vi "Word (Frame).vi"(8 "error in (no error)":errorcluster, 11 "Node Ptr":T2 format="%.0x") -> (0 "error out":errorcluster)   [LabVIEW 2020, in "Communication Bus Template System Explorer.lvlib" / "Implementation.lvlib"]
uses:
  Implementation.lvlib
  <vilib>/NI VeriStand/Custom Device API/Custom Device Item Ref.ctl
  <vilib>/NI VeriStand/Custom Device API/Custom Device API.lvlib
  Scripting/Communication Bus Template Scripting.lvlib
  Scripting/Constants.vi
  <vilib>/NI VeriStand/Custom Device API/Get Item Property (U16).vi
  <vilib>/NI VeriStand/Custom Device API/Get Item Property (Double).vi
  <vilib>/NI VeriStand/Custom Device API/Get Item Property (U32).vi
  <vilib>/NI VeriStand/Custom Device API/Get Item Property (Boolean).vi
panel:
  out "Transfer Type":T1(ring)
  out "SDI":u8 format="%o"
  out "SDI Enabled":bool
  out "Transfer Rate (Hz)":dbl
  out "Label (Octal)":i32 format="%o"
  out "Label (Decimal)":i32
  in  "SHDocVw.IWebBrowser":refnum<k7>(container)
  in  "Specific Header":cluster{"Section Name":string}={"Section Name"="Specific Page Settings"}
  in  "General Header":cluster{"Section Name":string}={"Section Name"="General Page Settings"}
  in  "Description":string
  in  "Name":string
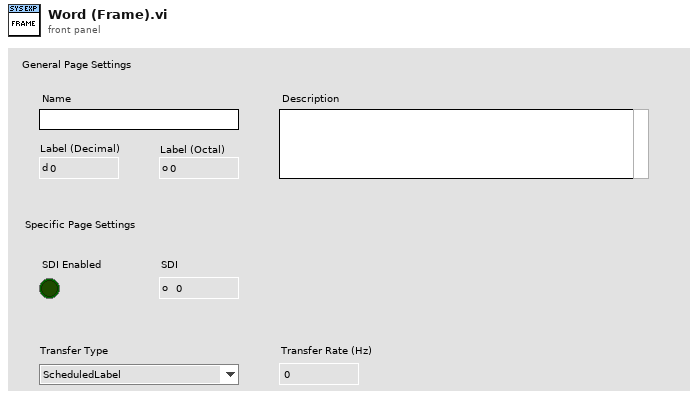
[diagram p1: front panel]
types:
  T1 = enum16{"ScheduledLabel", "Acyclic", "Block", "Strobe"}
  T2 = typedef "Custom Device API.lvlib/Custom Device Item Ref.ctl" = u64
  T3 = typedef "Custom Device API.lvlib/Custom Device Item Info.ctl" = cluster{"Name":string, "Is Channel":bool, "GUID":string, "Is Waveform":bool}
  T4 = typedef "Custom Device API.lvlib/Custom Device Commands.ctl" = enum16{"Default", "Item renamed", "Shutdown", "Dynamic button pressed"}
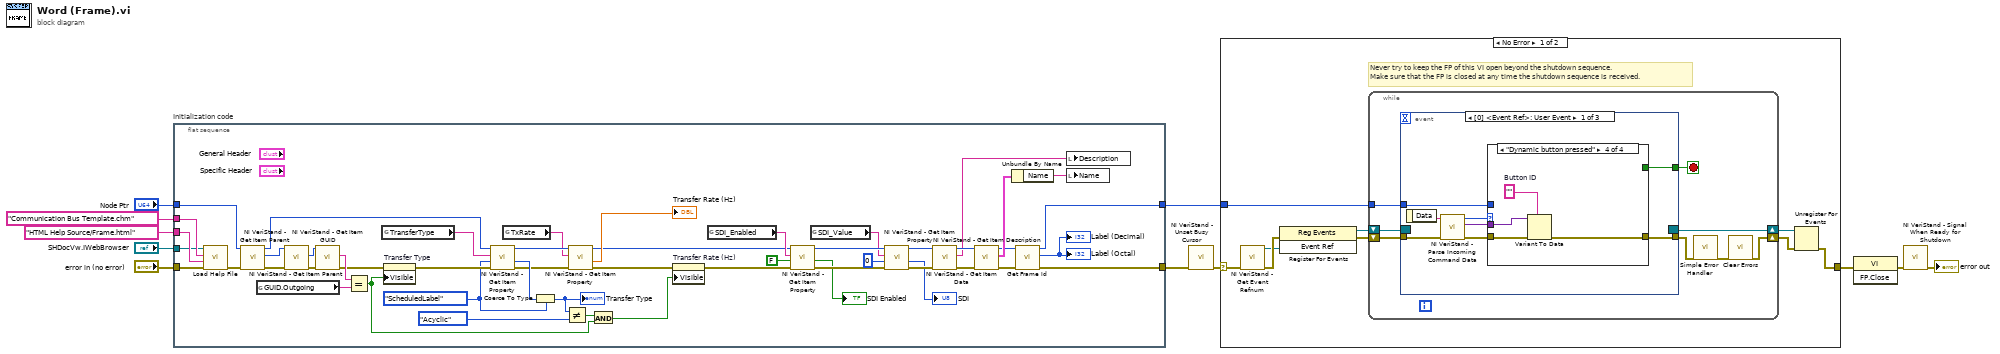
[diagram p0: block diagram]
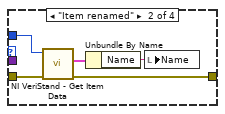
[diagram p3: hidden frame]
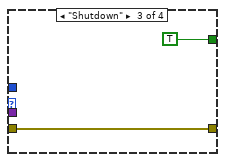
[diagram p4: hidden frame]
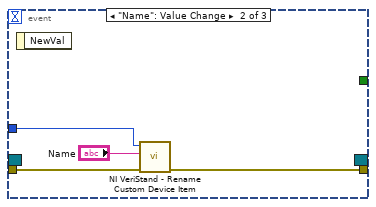
[diagram p5: hidden frame]
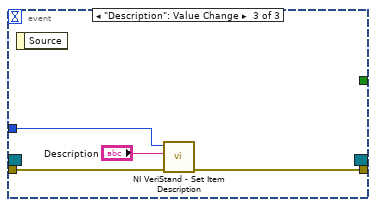
[diagram p6: hidden frame]
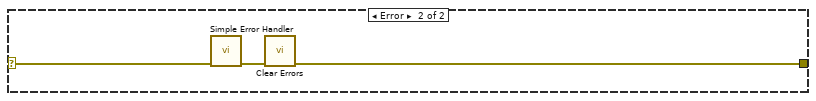
[diagram p7: hidden frame]
diagram:
  n1 = flat-sequence "Initialization code" {
    tunnel: "error in (no error)" -> [w55]
    tunnel: "Node Ptr" -> [w40]
    tunnel: [w49] -> w7
    tunnel: [w48] -> w4
    tunnel: "SHDocVw.IWebBrowser" -> [w52]
    tunnel: "HTML Help Source/Frame.html" ("CD_CHM_Section") -> [w54]
    tunnel: "Communication Bus Template.chm" ("CD_CHM_FileName") -> [w53]
    frame #0 {
      w35 = T1."ScheduledLabel" ("Transfer Type")
      n2 = call "Load Help File.vi"("error in (no error)"=w55, "HTML File to Load"=w54, "Main CHM File"=w53, "Browser"=w52) -> ("error out"=w41:errorcluster)  [unwired: 7 in]
      n3 = call <vilib>:"NI VeriStand - Get Item Parent.vi"("error in (no error)"=w41, "Item Ref in"=w40) -> ("error out"=w46:errorcluster, "Parent Ref"=w45:T2, "Item Ref out"=w36:T2)  [unwired: 6 in, 1 out]
      n4 = global read "Constants.vi" "GUID.Outgoing"() -> (w39:string)
      n5 = call <vilib>:"NI VeriStand - Get Item Parent.vi"("error in (no error)"=w46, "Item Ref in"=w45) -> ("error out"=w44:errorcluster, "Parent Ref"=w42:T2)  [unwired: 6 in, 2 out]
      n6 = call <vilib>:"NI VeriStand - Get Item GUID.vi"("error in (no error)"=w44, "Item Ref in"=w42) -> ("error out"=w38:errorcluster, "GUID"=w43:string)  [unwired: 7 in, 1 out]
      n7 = Equal?(x=w43, y=w39) -> (x = y?=w30:bool)
      n8 = global read "Constants.vi" "TransferType"() -> (w28:string)
      n9 = property on="Transfer Type" class="Enum (strict)"(error in=w38, "Visible"=w30) -> (error out=w37:errorcluster)  [unwired: 1 in, 1 out]
      n10 = call-poly <vilib>:"NI VeriStand - Get Item Property.vi"("error in (no error)"=w37, "Default Value"=w35, "Property Name"=w28, "Item Ref in"=w36) -> ("error out"=w27:errorcluster, "Value"=w34:u16, "Item Ref out"=w25:T2)  [unwired: 4 in, 1 out]
      n11 = global read "Constants.vi" "TxRate"() -> (w24:string)
      n12 = Coerce To Type(0:w34, 1:w35) -> (2:w33:T1)
      "Transfer Type" <- w33
      n13 = Not Equal?(x=w33, y=T1."Acyclic" ("Transfer Type")) -> (x != y?=w31:bool)
      n14 = call-poly <vilib>:"NI VeriStand - Get Item Property.vi"("error in (no error)"=w27, "Property Name"=w24, "Item Ref in"=w25) -> ("error out"=w26:errorcluster, "Value"=→"Transfer Rate (Hz)":dbl, "Item Ref out"=w17:T2)  [unwired: 5 in, 1 out]
      n15 = And(x=w31, y=w30) -> (x .and. y?=w29:bool)
      n16 = property on="Transfer Rate (Hz)" class="DigNum (strict)"(error in=w26, "Visible"=w29) -> (error out=w16:errorcluster)  [unwired: 1 in, 1 out]
      n17 = global read "Constants.vi" "SDI_Enabled"() -> (w18:string)
      n18 = call-poly <vilib>:"NI VeriStand - Get Item Property.vi"("error in (no error)"=w16, "Default Value"=FALSE, "Property Name"=w18, "Item Ref in"=w17) -> ("error out"=w19:errorcluster, "Value"=→"SDI Enabled":bool, "Item Ref out"=w20:T2)  [unwired: 4 in, 1 out]
      n19 = global read "Constants.vi" "SDI_Value"() -> (w15:string)
      n20 = call-poly <vilib>:"NI VeriStand - Get Item Property.vi"("error in (no error)"=w19, "Default Value"=u8 0 ("SDI"), "Property Name"=w15, "Item Ref in"=w20) -> ("Value"=→"SDI":u32, "Item Ref out"=w12:T2)  [unwired: 4 in, 2 out]
      n21 = call <vilib>:"NI VeriStand - Get Item Description.vi"("error in (no error)"=w16, "Item Ref in"=w12) -> ("error out"=w59:errorcluster, "Description"=w56:string, "Item Ref out"=w60:T2)  [unwired: 7 out]
      n22 = call <vilib>:"NI VeriStand - Get Item Data.vi"("error in (no error)"=w59, "Item Ref in"=w60) -> ("error out"=w50:errorcluster, "Item Info"=w58:T3, "Item Ref out"=w51:T2)  [unwired: 7 out]
      n23 = Unbundle By Name(w58) -> ("Name"=w57:string)
      n24 = call "Get Frame Id.vi"("error in"=w50, "Frame Ref"=w51) -> ("error out"=w49:errorcluster, "ID"=→"Label (Decimal)" →"Label (Octal)":i32, "Frame Ref out"=w48:T2)  [unwired: 7 in]
      n25 = local write "Description"(w56) -> ()
      n26 = local write "Name"(w57) -> ()
    }
  }
  n27 = call <vilib>:"NI VeriStand - Unset Busy Cursor.vi"("error in (no error)"=w7) -> ("error out"=w6:errorcluster)  [unwired: 10 out]
  n28 = case shown="No Error" w6 {
    selector: w6 -> [w61 w108]
    tunnel: [w66 w106] -> w11
    tunnel: w4 -> [w62 _]
    frame No Error {
      # "Never try to keep the FP of this VI open beyond the shutdown sequence.\nMake sure that the FP is closed at any time the shutdown sequence is received."
      n29 = call <vilib>:"NI VeriStand - Get Event Refnum.vi"("error in (no error)"=w61) -> ("error out"=w69:errorcluster, "Event Ref"=w65:refnum<user-event>)  [unwired: 9 out]
      n30 = register-events(error in=w69, w65) -> (reference out=w63:refnum<event-registration>, error out=w64:errorcluster)  [unwired: 1 in]
      n31 = while {
        tunnel: w62 -> [w73]
        shift-right: [w70] -> w67
        shift-left: w64 -> [w76]
        shift-right: [w77] -> w68
        shift-left: w63 -> [w75]
        stop <- w74 stop-if-true
        n32 = event shown="[0] <Event Ref>: User Event" {
          selector: w75 -> [_ _ _]
          dyn-events: [_ _ _] -> w77
          timeout: _ -> [_ _ _]
          tunnel: w76 -> [w85 w101 w104]
          tunnel: [w81 _ _] -> w74
          tunnel: [w80 w100 w103] -> w72
          tunnel: w73 -> [w79 w99 w105]
          event User Event {
            n33 = event-data() -> ("Data"=w84:string)  [unwired: 1 out]
            n34 = call <vilib>:"NI VeriStand - Parse Incoming Command Data.vi"("error in (no error)"=w85, "Incoming data"=w84) -> ("error out"=w83:errorcluster, "Outgoing data"=w78:variant, "Action"=w82:T4)  [unwired: 7 out]
            n35 = case shown="\"Dynamic button pressed\"" w82 {
              tunnel: w83 -> [w86 w91 w92 w97]
              tunnel: [_ _ TRUE _] -> w81
              tunnel: [w86 w88 w92 w94] -> w80
              tunnel: w79 -> [_ w90 _ _]
              tunnel: w78 -> [_ _ _ w96]
              frame "Default", Default {
              }
              frame "Item renamed" {
                n36 = call <vilib>:"NI VeriStand - Get Item Data.vi"("error in (no error)"=w91, "Item Ref in"=w90) -> ("error out"=w88:errorcluster, "Item Info"=w89:T3)  [unwired: 8 out]
                n37 = Unbundle By Name(w89) -> ("Name"=w87:string)
                n38 = local write "Name"(w87) -> ()
              }
              frame "Shutdown" {
              }
              frame "Dynamic button pressed" {
                w95 = ""  # Button ID
                n39 = Variant To Data(error in=w97, type=w95, Variant=w96) -> (error out=w94:errorcluster)  [unwired: 1 out]
              }
            }
          }
          event "Name": Value Change {
            n40 = event-data() -> ()  [unwired: 2 out]
            n41 = call <vilib>:"NI VeriStand - Rename Custom Device Item.vi"("error in (no error)"=w101, "New Name"="Name", "Item Ref in"=w99) -> ("error out"=w100:errorcluster)  [unwired: 1 in, 7 out]
          }
          event "Description": Value Change {
            n42 = event-data() -> ()  [unwired: 2 out]
            n43 = call <vilib>:"NI VeriStand - Set Item Description.vi"("error in (no error)"=w104, "Description"="Description", "Item Ref in"=w105) -> ("error out"=w103:errorcluster)  [unwired: 8 out]
          }
        }
        n44 = call <vilib>:"Simple Error Handler.vi"("error in (no error)"=w72) -> ("error out"=w71:errorcluster)  [unwired: 1 in, 7 out]
        n45 = call <vilib>:"Clear Errors.vi"("error in (no error)"=w71) -> ("error out"=w70:errorcluster)  [unwired: 1 in, 5 out]
      }
      n46 = Unregister For Events(event registration refnum=w68, error in=w67) -> (error out=w66:errorcluster)
    }
    frame Error {
      n47 = call <vilib>:"Simple Error Handler.vi"("error in (no error)"=w108) -> ("error out"=w107:errorcluster)  [unwired: 1 in, 7 out]
      n48 = call <vilib>:"Clear Errors.vi"("error in (no error)"=w107) -> ("error out"=w106:errorcluster)  [unwired: 1 in, 5 out]
    }
  }
  n49 = invoke class="VI" method="FP.Close"(error in=w11) -> (error out=w10:errorcluster)  [unwired: 2 in, 2 out]
  n50 = call <vilib>:"NI VeriStand - Signal When Ready for Shutdown.vi"("error in (no error)"=w10) -> ("error out"=→"error out":errorcluster)  [unwired: 10 out]
